vi "acquireValue.vi"(8 "error in (no error)":errorcluster, 10 "nextSample?":bool, 11 "stopMotionAllAxis in":refnum<class "stopMotionAllAxis.lvclass">) -> (0 "error out":errorcluster, 1 "function return":i32, 2 "variantData":variant, 3 "stopMotionAllAxis out":refnum<class "stopMotionAllAxis.lvclass">)   [LabVIEW 2016, in "SALLV_AtDome_Messaging.lvlib" / "stopMotionAllAxis.lvclass"]
uses:
  stopMotionAllAxis.lvclass
  ts_sallv_AtDome/SALLV_AtDome.lvlib
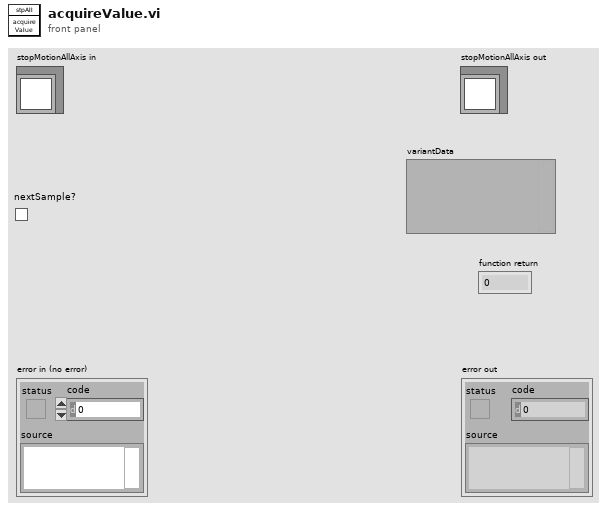
[diagram p1: front panel]
types:
  T1 = typedef "SALLV_AtDome.lvlib/command_stopMotionAllAxis.ctl" = cluster{"value":bool}
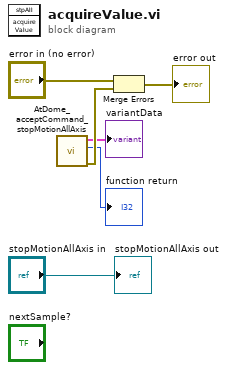
[diagram p0: block diagram]
diagram:
  n1 = call "AtDome_acceptCommand_stopMotionAllAxis.vi"() -> ("error out"=w3:errorcluster, "function return"=→"function return":i32, "command_stopMotionAllAxis_Ctl out"=→"variantData":T1)  [unwired: 9 in]
  n2 = Merge Errors("error in (no error)", w3) -> (→"error out":errorcluster)
  "stopMotionAllAxis out" <- "stopMotionAllAxis in"
